vi "Queue Reference (library variable).vi"() -> ()   [LabVIEW 2016, in "Anti-Spam Tester (AST).lvlib" / "AST MHL Queue.lvclass"]
uses:
  AST MHL Queue.lvclass
  Command (enum).ctl
  Message (cluster).ctl
panel:
  in  "Queue Reference":refnum<queue>
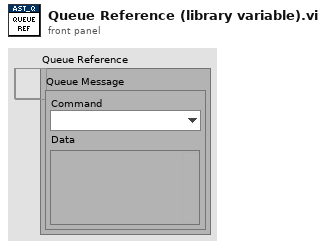
[diagram p1: front panel]
diagram:
